vi "Demo v2.vi"() -> ()   [LabVIEW 2013]
panel:
  out "SCORE":i32
  out "FAIL!":bool
  in  "a":dbl=-0.3
  in  "Jump speed":dbl=3.0
  in  "Jump":bool
  out "Picture":i32[][](graph)
  in  "stop":bool
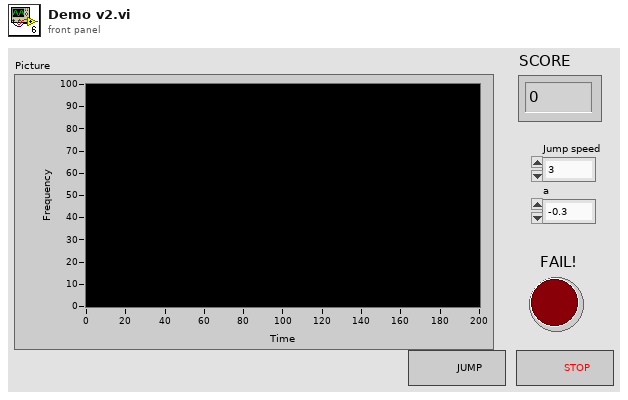
[diagram p1: front panel]
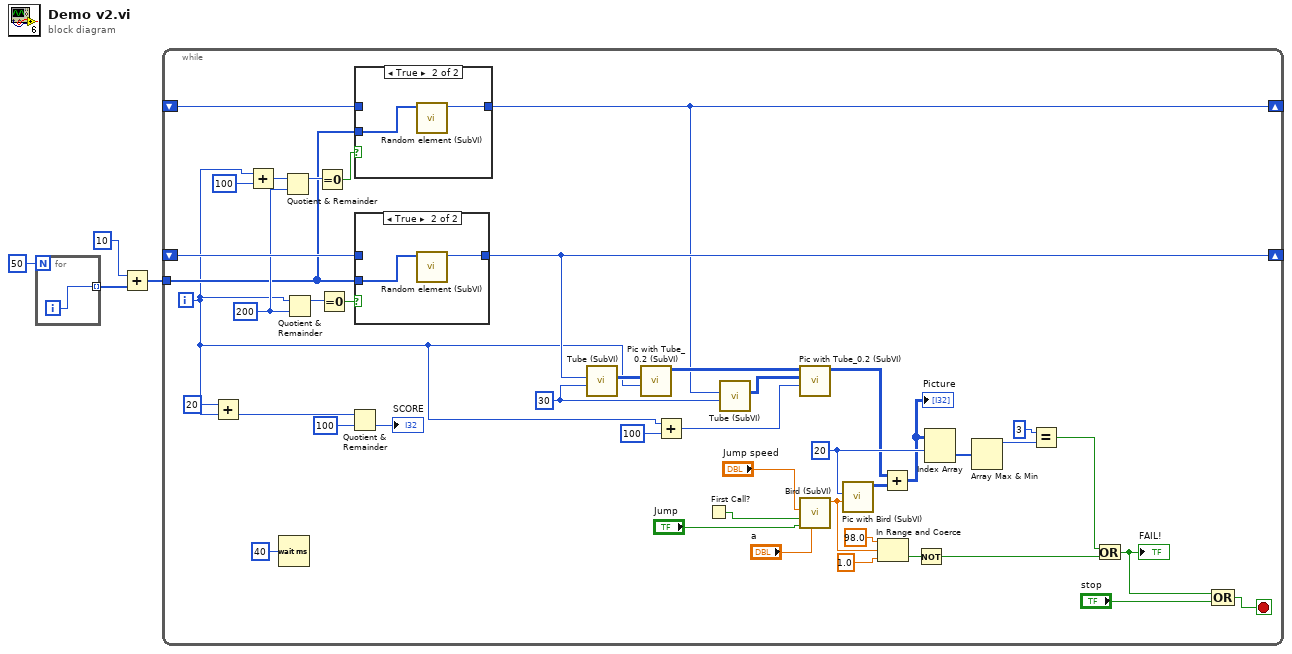
[diagram p0: block diagram]
diagram:
  n1 = for {
    N: 50 -> [_]
    tunnel: [w5] -> w3 mode=indexing
    i -> [w5]
  }
  n2 = Add(x=10, y=w3) -> (x+y=w1:i32[])
  n3 = while {
    tunnel: w1 -> [w19]
    shift-right: [w26] -> _
    shift-left: _ -> [w27]
    shift-right: [w18] -> _
    shift-left: _ -> [w20]
    i -> [w11]
    stop <- w41 stop-if-true
    w22 = 200 ("y")
    w33 = 20 ("X position")
    w42 = 30 ("Gap height (30)")
    n4 = Add(x=20, y=w11) -> (x+y=w7:i32)
    n5 = Add(x=w11, y=100) -> (x+y=w23:i32)
    n6 = Wait (ms)(milliseconds to wait=u32 40) -> ()  [unwired: 1 out]
    n7 = Quotient & Remainder(x=w23, y=w22) -> (x-y*floor(x/y)=w24:i32)  [unwired: 1 out]
    n8 = Quotient & Remainder(x=w11, y=w22) -> (x-y*floor(x/y)=w29:i32)  [unwired: 1 out]
    n9 = Equal To 0?(x=w24) -> (x = 0?=w21:bool)
    n10 = Equal To 0?(x=w29) -> (x = 0?=w28:bool)
    n11 = Quotient & Remainder(x=w7, y=100) -> (floor(x/y)=→"SCORE":i32)  [unwired: 1 out]
    n12 = case shown="True" w21 {
      tunnel: [w50 w52] -> w18
      tunnel: w20 -> [w50 _]
      tunnel: w19 -> [_ w51]
      frame False {
      }
      frame True {
        n13 = call "Random element (SubVI).vi"("Array"=w51) -> ("random element"=w52:i32)  [unwired: 10 in]
      }
    }
    n14 = case shown="True" w28 {
      tunnel: [w53 w55] -> w26
      tunnel: w27 -> [w53 _]
      tunnel: w19 -> [_ w54]
      frame False {
      }
      frame True {
        n15 = call "Random element (SubVI).vi"("Array"=w54) -> ("random element"=w55:i32)  [unwired: 10 in]
      }
    }
    n16 = call "Tube (SubVI).vi"("Gap height (30)"=w42, "Gap low y"=w26) -> ("Tube"=w44:i32[][])  [unwired: 9 in]
    n17 = call "Pic with Tube_0.2 (SubVI).vi"("Tube x"=w11, "Tube"=w44) -> ("Picture"=w43:i32[][])  [unwired: 9 in]
    n18 = Add(x=w11, y=100) -> (x+y=w9:i32)
    n19 = First Call?() -> (First Call?: T/F=w8:bool)
    n20 = call "Tube (SubVI).vi"("Gap height (30)"=w42, "Gap low y"=w18) -> ("Tube"=w13:i32[][])  [unwired: 9 in]
    n21 = call "Pic with Tube_0.2 (SubVI).vi"("Tube x"=w9, "Tube"=w13, "Picture in"=w43) -> ("Picture"=w12:i32[][])  [unwired: 8 in]
    n22 = call "Bird (SubVI).vi"("a"="a", "Jump"="Jump", "Reset"=w8, "Jump speed"="Jump speed") -> ("Position"=w40:dbl)  [unwired: 7 in]
    n23 = call "Pic with Bird (SubVI).vi"("Bird Position"=w40, "X position"=w33) -> ("Picture"=w47:i32[][])  [unwired: 9 in]
    n24 = In Range and Coerce(upper limit=98.0, x=w40, lower limit=1.0) -> (In Range?=w37:bool)  [unwired: 1 out]
    n25 = Add(x=w12, y=w47) -> (x+y=w32:i32[][])
    "Picture" <- w32
    n26 = Not(x=w37) -> (.not. x?=w31:bool)
    n27 = Index Array(array=w32, index (row)=w33) -> (element=w36:i32[])  [unwired: 1 in]
    n28 = Array Max & Min(array=w36) -> (max value=w35:i32)  [unwired: 3 out]
    n29 = Equal?(x=3 ("y"), y=w35) -> (x = y?=w30:bool)
    n30 = Or(x=w30, y=w31) -> (x .or. y?=w15:bool)
    "FAIL!" <- w15
    n31 = Compound Arithmetic op=OR(w15, "stop") -> (w41:bool)
  }
